vi "Notify Task Completed.vi"(8 "error in (no error)":errorcluster, 11 "Device in":refnum<class "Device.lvclass">) -> (0 "error out":errorcluster, 3 "Device out":refnum<class "Device.lvclass">)   [LabVIEW 2023, in "Device.lvlib" / "Device.lvclass"]
uses:
  Device.lvclass
  Device.lvclass/Device.ctl
  <vilib>/ActorFramework/Actor/Actor.lvclass
  Application Messages/Automation_TaskCompleted Msg/Automation_TaskCompleted Msg.lvclass
  C:/Program Files/National Instruments/LabVIEW 2023/vi.lib/ActorFramework/Actor/Actor.lvclass
  C:/FlashGordon/Development/Hardware/Device/Device.lvclass
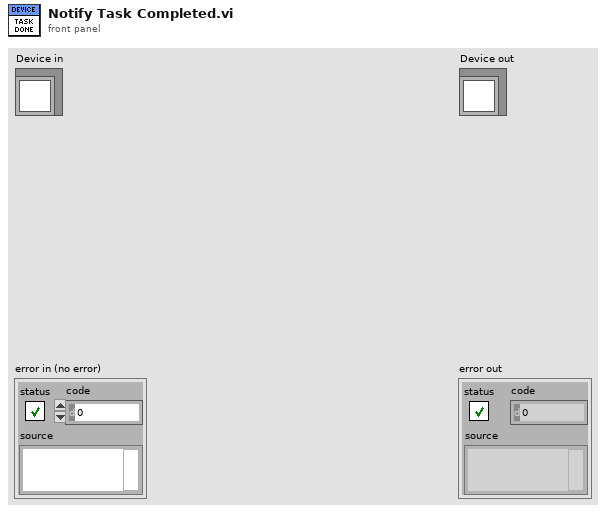
[diagram p1: front panel]
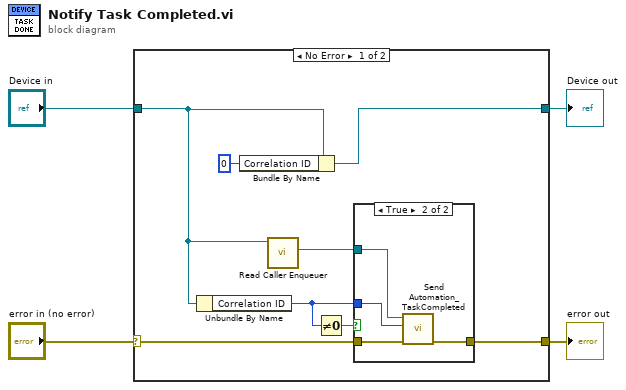
[diagram p0: block diagram]
diagram:
  n1 = case shown="No Error" "error in (no error)" {
    selector: "error in (no error)" -> [w12 w19]
    tunnel: [w11 w19] -> w3
    tunnel: [w8 w18] -> w1
    tunnel: "Device in" -> [w9 w18]
    frame No Error {
      n2 = Unbundle By Name(w9) -> ("Correlation ID"=w6:u32)
      n3 = Bundle By Name(cluster=w9, "Correlation ID"=u32 0) -> (w8:refnum<class "Device.lvclass">)
      n4 = call <vilib>:"Read Caller Enqueuer.vi"("Actor"=w9) -> ("Caller Enqueuer"=w10:refnum<class "Message Enqueuer.lvclass">)  [unwired: 10 in]
      n5 = Not Equal To 0?(x=w6) -> (x != 0?=w5:bool)
      n6 = case shown="True" w5 {
        tunnel: w12 -> [w13 w17]
        tunnel: [w13 w16] -> w11
        tunnel: w10 -> [_ w15]
        tunnel: w6 -> [_ w14]
        frame False {
        }
        frame True {
          n7 = call "Send Automation_TaskCompleted.vi"("error in (no error)"=w17, "Correlation ID"=w14, "Message Enqueuer"=w15) -> ("error out"=w16:errorcluster)  [unwired: 7 in, 1 out]
        }
      }
    }
    frame Error {
    }
  }
  "error out" <- w3
  "Device out" <- w1
